vi "Wait.vi"(0 "Data Task in":refnum<k21>, 1 "PS type":enum16{"NHR", "ITECH"}(ring), 5 "data task error in":errorcluster, 7 "#DAQ outputs (1-13)":i32, 9 "PS VISA in":refnum<visa-resource-name>, 11 "PS error in":errorcluster caption="PS error in (no error)", 12 "Wait Filepath":path=path "C:/Users/ga11/Desktop/VI/results/3PtestChrgRest.lvm" caption="Filename", 13 "Wait time":dbl) -> (4 "data task out":refnum<k21>, 6 "data task error out":errorcluster, 10 "PS Visa Out":refnum<visa-resource-name>, 15 "PS error out":errorcluster)   [LabVIEW 2020]
uses:
  Drivers-Essentials/Read (Ave Current).vi
  Drivers-NHR-9200/NHR/Public/Data/Low Level/Fetch (Ave Voltage).vi
  Drivers-Essentials/NH Research Regenerative Test Series.lvlib
  Drivers-IT-M3400/IT-M3400.lvlib
panel:
  out "Ave Current (A)":dbl
  out "Ave Voltage (V)":dbl
  out "WaitElapsed Time (s)":i32 caption="Elapsed Time (s)"
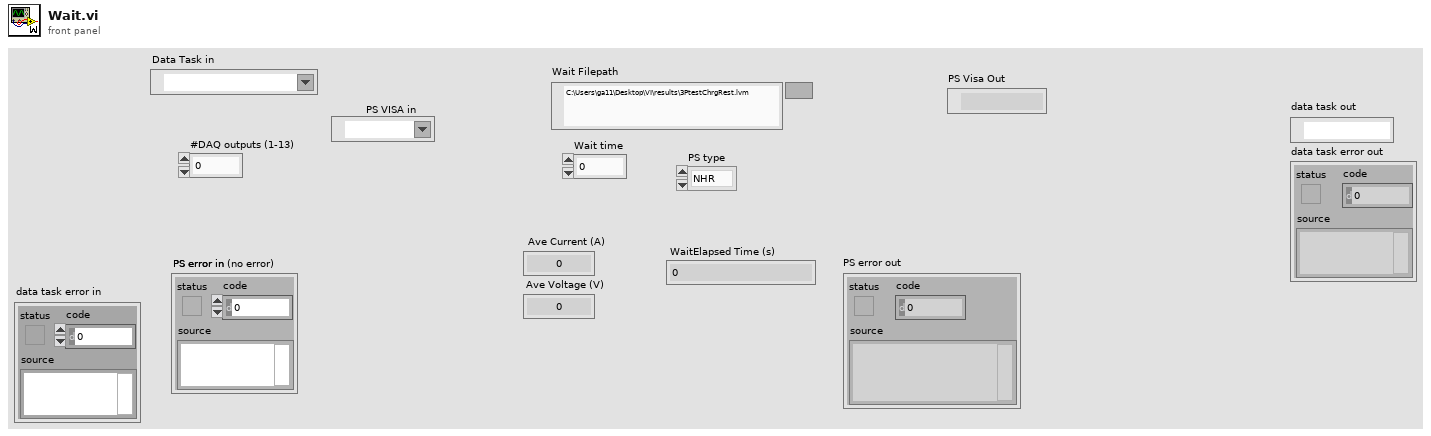
[diagram p1: front panel]
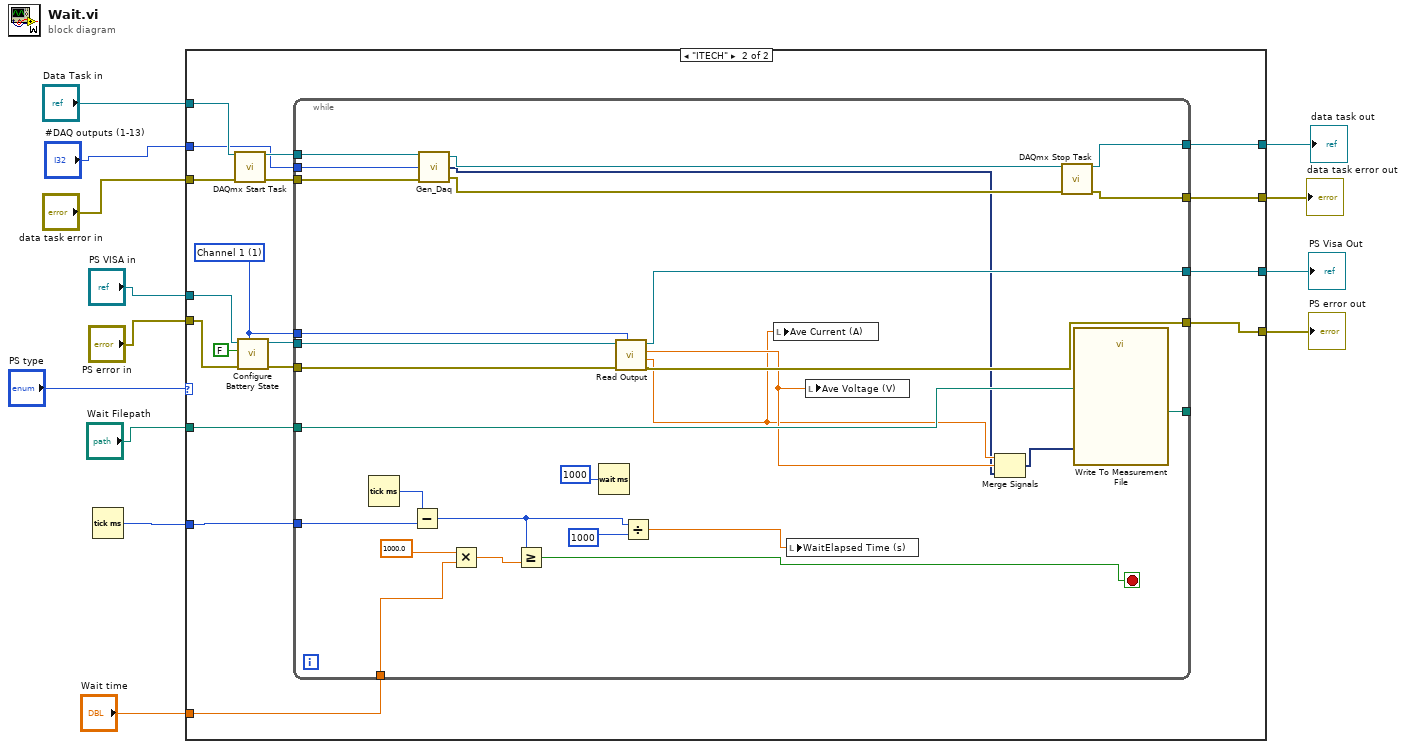
[diagram p0: block diagram]
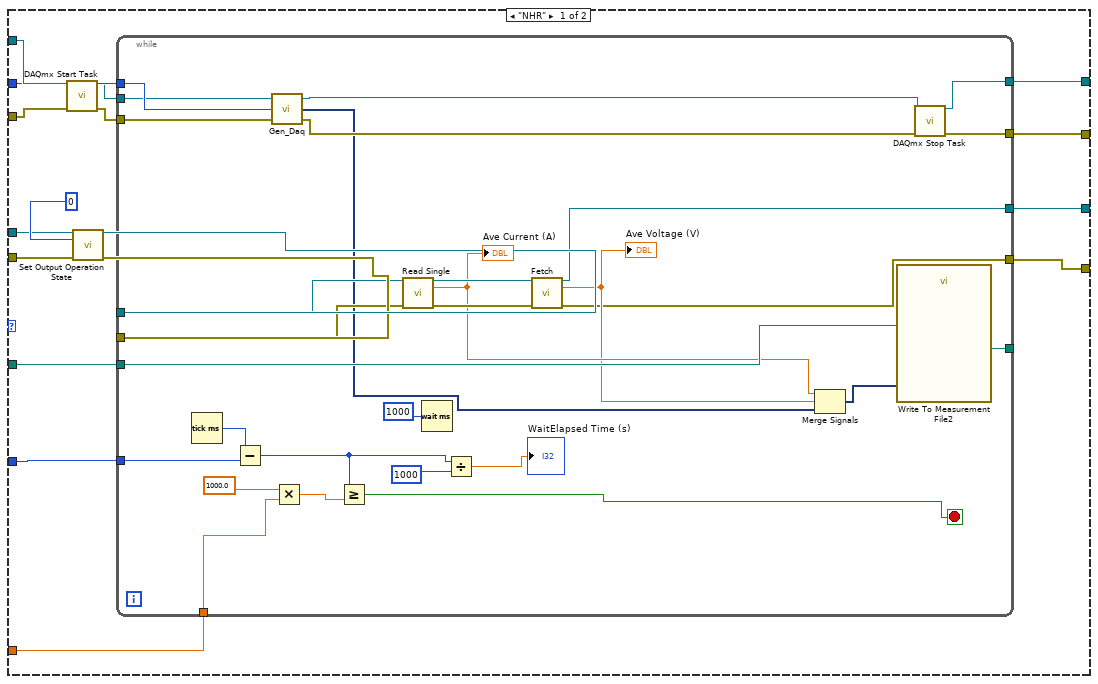
[diagram p2: hidden frame]
diagram:
  n1 = Tick Count (ms)() -> (millisecond timer value=w12:u32)
  n2 = case shown="\"ITECH\"" "PS type" {
    tunnel: "Wait time" -> [w27 w77]
    tunnel: w12 -> [w26 w76]
    tunnel: "PS VISA in" -> [w25 w70]
    tunnel: "PS error in" -> [w24 w69]
    tunnel: "Wait Filepath" -> [w23 w75]
    tunnel: [w22 w74] -> w8
    tunnel: [w21 w73] -> w7
    tunnel: "Data Task in" -> [w20 w66]
    tunnel: "data task error in" -> [w19 w65]
    tunnel: "#DAQ outputs (1-13)" -> [w18 w62]
    tunnel: [w15 w61] -> w2
    tunnel: [w14 w60] -> w1
    frame "NHR" {
      n3 = call <vilib>:"DAQmx Start Task.vi"("task/channels in"=w20, "error in"=w19) -> ("task out"=w17:refnum<k21>, "error out"=w16:errorcluster)  [unwired: 12 in]
      n4 = call "Set Output Operation State.vi"("VISA resource name"=w25, "Mode (0: Off)"=0, "error in (no error)"=w24) -> ("VISA resource name out"=w29:refnum<visa-resource-name>, "error out"=w28:errorcluster)  [unwired: 11 in]
      n5 = while {
        tunnel: w29 -> [w57]
        tunnel: w28 -> [w56]
        tunnel: w27 -> [w52]
        tunnel: [w49] -> _
        tunnel: w26 -> [w48]
        tunnel: w23 -> [w47]
        tunnel: [w40] -> w22
        tunnel: [w39] -> w21
        tunnel: w18 -> [w36]
        tunnel: w17 -> [w35]
        tunnel: w16 -> [w34]
        tunnel: [w33] -> w15
        tunnel: [w32] -> w14
        stop <- w53 stop-if-true
        n6 = Tick Count (ms)() -> (millisecond timer value=w54:u32)
        n7 = Subtract(x=w54, y=w48) -> (x-y=w46:u32)
        n8 = call "Gen_Daq.vi"("error in"=w34, "#DAQ outputs (1-13)"=w36, "task/channels in"=w35) -> ("error out"=w37:errorcluster, "DaQ_output"=w31:dynamicdata, "task out"=w38:refnum<k21>)
        n9 = Multiply(x=1000.0, y=w52) -> (x*y=w50:dbl)
        n10 = Greater Or Equal?(x=w46, y=w50) -> (x >= y?=w53:bool)
        n11 = call-poly "Read Single.vi"("VISA resource name"=w57, "error in (no error)"=w56) -> ("VISA resource name out"=w58:refnum<visa-resource-name>, "Ave Current (A)"=w43:dbl, "error out"=w59:errorcluster)  [unwired: 11 in]
        "Ave Current (A)" <- w43
        n12 = Wait (ms)(milliseconds to wait=1000) -> ()  [unwired: 1 out]
        n13 = Divide(x=w46, y=1000) -> (x/y=→"WaitElapsed Time (s)":dbl)
        n14 = call-poly "Fetch.vi"("VISA resource name"=w58, "error in (no error)"=w59) -> ("VISA resource name out"=w40:refnum<visa-resource-name>, "Ave Voltage (V)"=w41:dbl, "error out"=w39:errorcluster)  [unwired: 11 in]
        "Ave Voltage (V)" <- w41
        n15 = Merge Signals "Merge Signals"(w43, w41, w31) -> (w42:dynamicdata)
        n16 = call "Write To Measurement File2"("Signals"=w42, "Filename"=w47) -> ("Filename Out"=w49:path)  [unwired: 15 in, 2 out]
        n17 = call <vilib>:"DAQmx Stop Task.vi"("task/channels in"=w38, "error in"=w37) -> ("task out"=w33:refnum<k21>, "error out"=w32:errorcluster)  [unwired: 12 in]
      }
    }
    frame "ITECH" {
      w67 = 1 items=["Channel 1"=1, "Channel 2"=2, "Channel 3"=3, "Channel 4"=4, "Channel 5"=5, "Channel 6"=6, "Channel 7"=7, "Channel 8"=8, "Channel 8"=9, "Channel 10"=10, "Channel 11"=11, "Channel 12"=12, "Channel 13"=13, "Channel 14"=14, "Channel 15"=15, "Channel 16"=16] ("Channel")
      n18 = call <vilib>:"DAQmx Start Task.vi"("task/channels in"=w66, "error in"=w65) -> ("task out"=w64:refnum<k21>, "error out"=w63:errorcluster)  [unwired: 12 in]
      n19 = call "Configure Battery State.vi"("Channel"=w67, "error in"=w69, "State"=FALSE, "VISA resource name"=w70) -> ("error out"=w71:errorcluster, "VISA resource name out"=w72:refnum<visa-resource-name>)  [unwired: 6 in]
      n20 = while {
        tunnel: w77 -> [w102]
        tunnel: [w99] -> _
        tunnel: w76 -> [w98]
        tunnel: w75 -> [w97]
        tunnel: [w93] -> w74
        tunnel: [w92] -> w73
        tunnel: w72 -> [w88]
        tunnel: w71 -> [w87]
        tunnel: w67 -> [w86]
        tunnel: w64 -> [w85]
        tunnel: w63 -> [w84]
        tunnel: w62 -> [w83]
        tunnel: [w80] -> w61
        tunnel: [w79] -> w60
        stop <- w103 stop-if-true
        n21 = Tick Count (ms)() -> (millisecond timer value=w104:u32)
        n22 = Subtract(x=w104, y=w98) -> (x-y=w96:u32)
        n23 = call "Gen_Daq.vi"("error in"=w84, "#DAQ outputs (1-13)"=w83, "task/channels in"=w85) -> ("error out"=w81:errorcluster, "DaQ_output"=w78:dynamicdata, "task out"=w82:refnum<k21>)
        n24 = Multiply(x=1000.0, y=w102) -> (x*y=w100:dbl)
        n25 = Greater Or Equal?(x=w96, y=w100) -> (x >= y?=w103:bool)
        n26 = Wait (ms)(milliseconds to wait=1000) -> ()  [unwired: 1 out]
        n27 = call "Read Output.vi"("Channel"=w86, "error in"=w87, "VISA resource name"=w88) -> ("error out"=w92:errorcluster, "Read Current(A)"=w90:dbl, "Read Voltage(V)"=w91:dbl, "VISA resource name out"=w93:refnum<visa-resource-name>)  [unwired: 5 in]
        n28 = Divide(x=w96, y=1000) -> (x/y=w89:dbl)
        n29 = local write "Ave Current (A)"(w90) -> ()
        n30 = local write "WaitElapsed Time (s)"(w89) -> ()
        n31 = local write "Ave Voltage (V)"(w91) -> ()
        n32 = Merge Signals "Merge Signals"(w90, w91, w78) -> (w94:dynamicdata)
        n33 = call <vilib>:"DAQmx Stop Task.vi"("task/channels in"=w82, "error in"=w81) -> ("task out"=w80:refnum<k21>, "error out"=w79:errorcluster)  [unwired: 12 in]
        n34 = call "Write To Measurement File"("Signals"=w94, "Filename"=w97) -> ("Filename Out"=w99:path)  [unwired: 15 in, 2 out]
      }
    }
  }
  "PS Visa Out" <- w8
  "PS error out" <- w7
  "data task out" <- w2
  "data task error out" <- w1
